vi "LVCAM Create Nest.vi"(9 "Alias":string, 10 "Nest Actor":refnum<class "LVCAM.lvclass">, 11 "Process in":refnum<class "ABD.lvclass">) -> (0 "error out":errorcluster, 3 "Process out":refnum<class "ABD.lvclass">)   [LabVIEW 2021, in "ABD.lvlib" / "ABD.lvclass"]
uses:
  ABD.lvclass
  LVCAM/LVCAM/LVCAM/LVCAM.lvclass
  ABD.lvclass/ABD.ctl
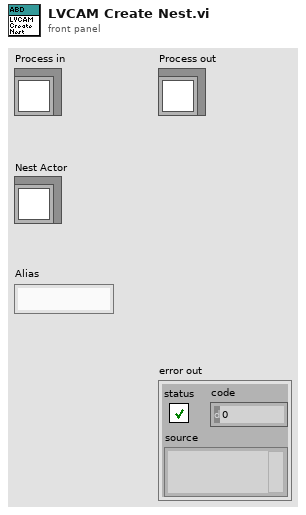
[diagram p1: front panel]
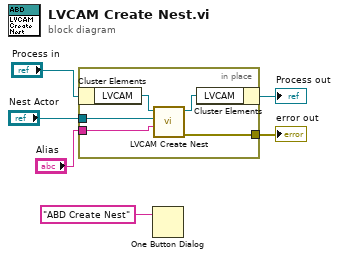
[diagram p0: block diagram]
diagram:
  n1 = in-place {
    in-place-border: "Nest Actor" -> [w9]
    in-place-border: "Alias" -> [w8]
    in-place-border: [w7] -> w3
    n2 = in-place-cluster #1("Process in") -> ("LVCAM"=w11:refnum<class "LVCAM.lvclass">)
    n3 = call-dynamic "LVCAM Create Nest.vi"("Alias"=w8, "Nest Actor"=w9, "LVCAM Create Nest in"=w11) -> ("error out"=w7:errorcluster, "LVCAM Create Nest out"=w10:refnum<class "LVCAM.lvclass">)  [unwired: 7 in]
    n4 = in-place-cluster #1("LVCAM"=w10) -> (→"Process out":refnum<class "ABD.lvclass">)
  }
  "error out" <- w3
  n5 = One Button Dialog(message="ABD Create Nest") -> ()  [unwired: 1 in, 1 out]
